vi "Log_File_Edits.vi"(0 "Job Directory":path=path "/G4_2_HD/Users/paulhayden/Documents/Projects/Hong Roughness/XW data/XW_Corr.tpt", 1 "File Editted?":bool, 2 "Channels to Edit":string[](array[string]), 3 "Data":string[][](array[string]), 4 "Results file name":path) -> ()   [LabVIEW 2011]
uses:
  Data_File_Type.ctl
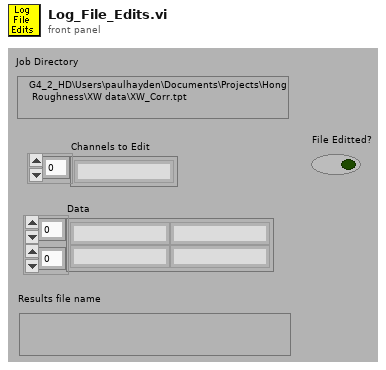
[diagram p1: front panel]
types:
  T1 = typedef "Data_File_Type.ctl" = enum16{"Read All File Types", "Results Files Only", "Raw Data Files Only", "Calibration Files Only", "Gas Desk Files Only", "Old Results Files Only", "Tabulated Data Files Only"}
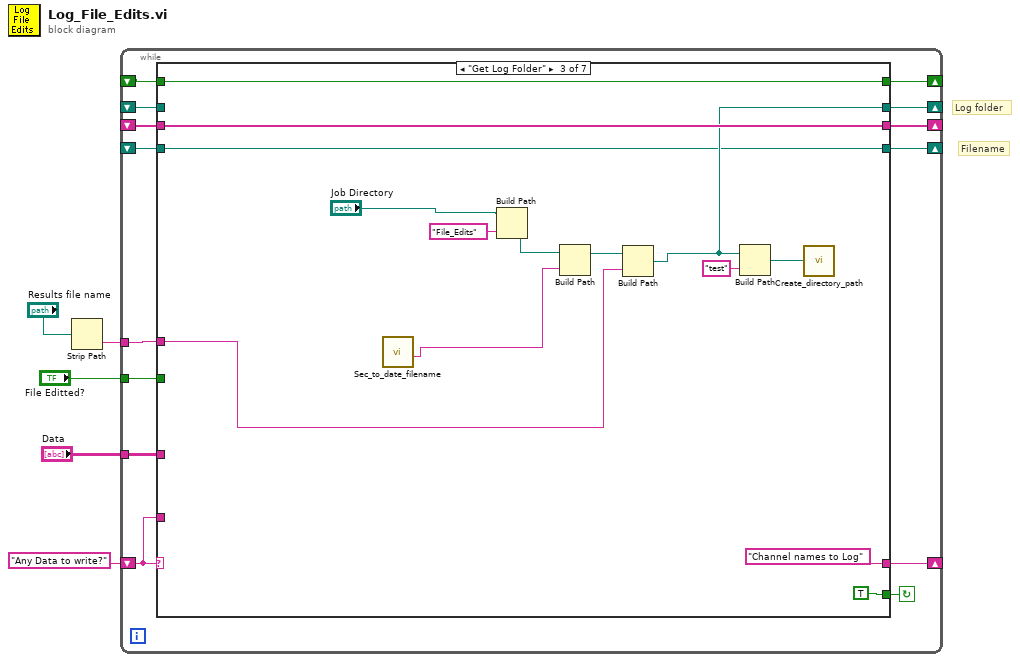
[diagram p0: block diagram]
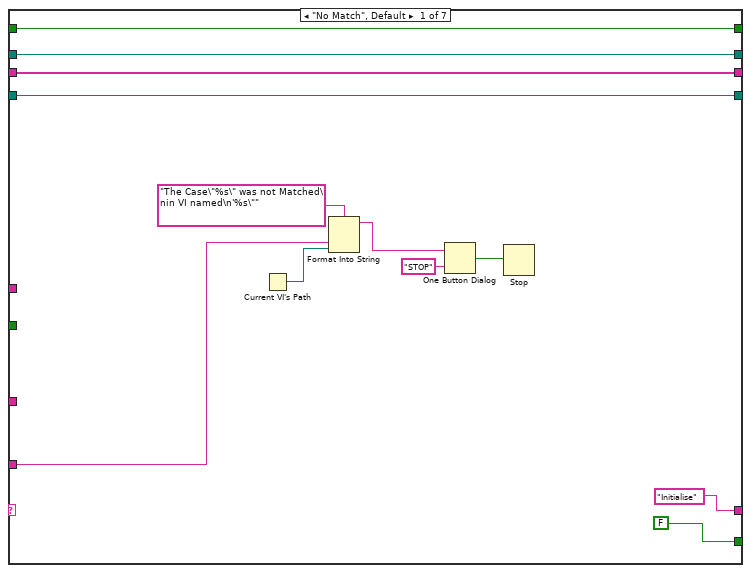
[diagram p2: hidden frame]
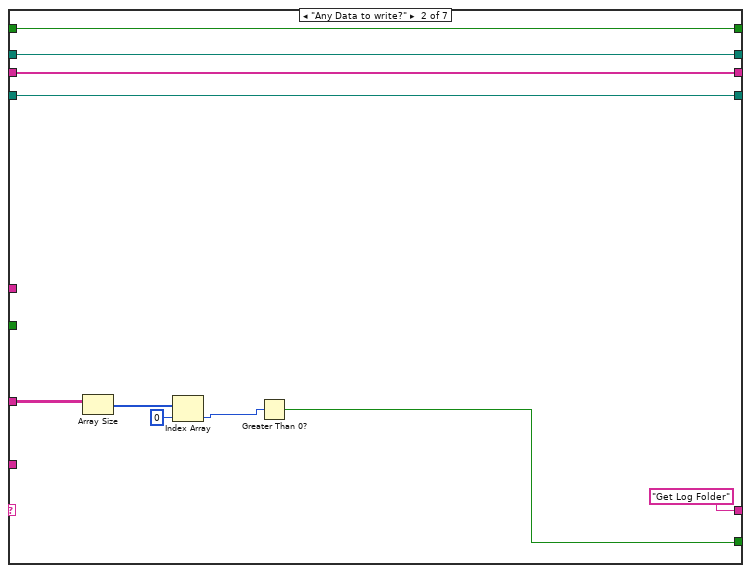
[diagram p3: hidden frame]
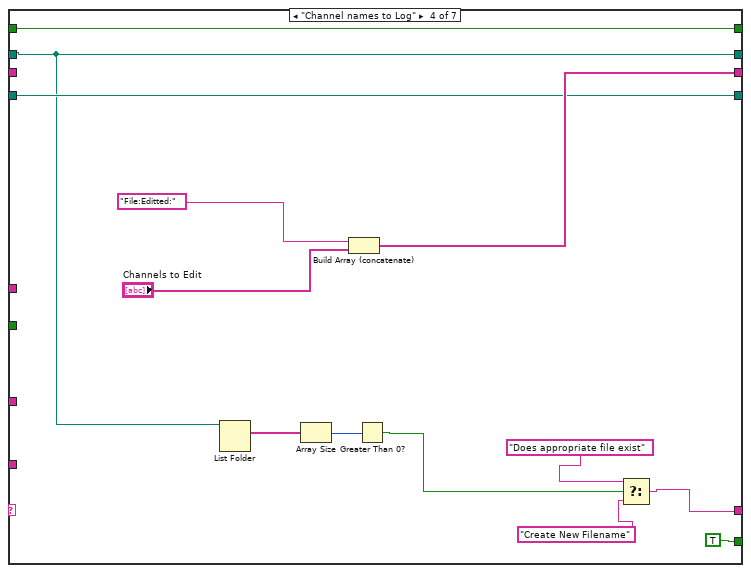
[diagram p4: hidden frame]
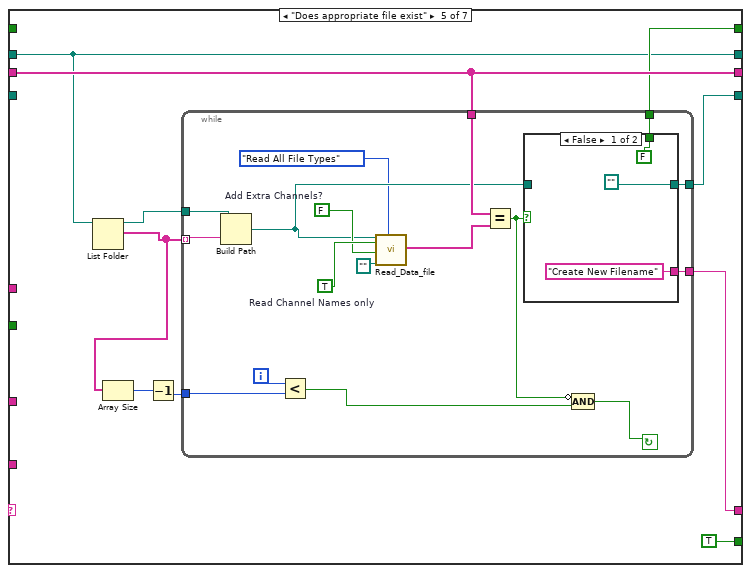
[diagram p5: hidden frame]
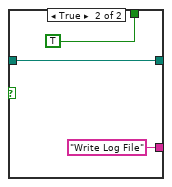
[diagram p6: hidden frame]
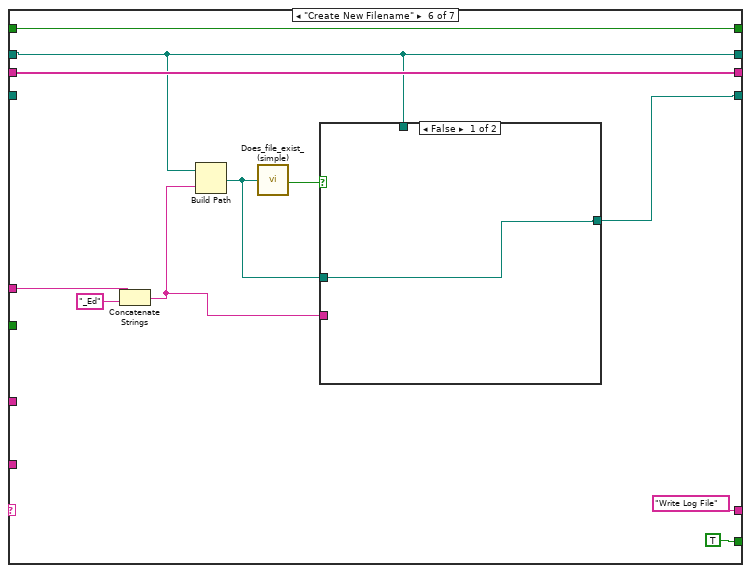
[diagram p7: hidden frame]
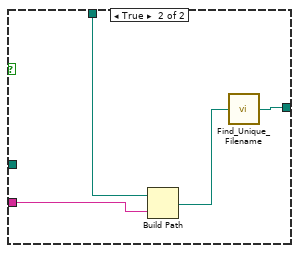
[diagram p8: hidden frame]
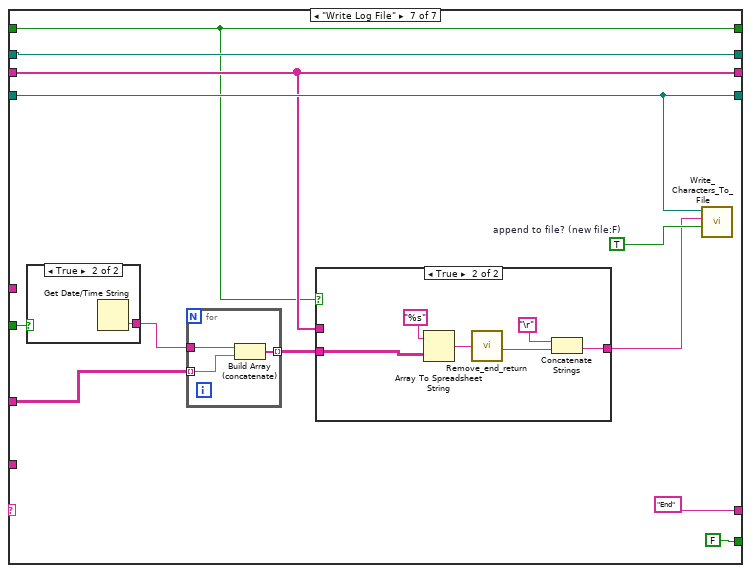
[diagram p9: hidden frame]
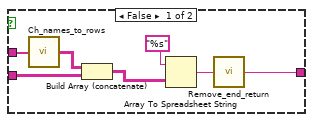
[diagram p10: hidden frame]
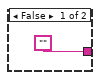
[diagram p11: hidden frame]
diagram:
  # "Filename"
  # "Log folder"
  n1 = Strip Path(path="Results file name") -> (name=w3:string)  [unwired: 1 out]
  n2 = while {
    shift-left: "Any Data to write?" -> [w17]
    shift-right: [w18] -> _
    shift-right: [w15] -> _
    shift-left: _ -> [w14]
    shift-right: [w16] -> _
    shift-left: _ -> [w13]
    tunnel: w3 -> [w12]
    shift-right: [w11] -> _
    shift-left: _ -> [w10]
    shift-right: [w9] -> _
    shift-left: _ -> [w8]
    tunnel: "File Editted?" -> [w7]
    tunnel: "Data" -> [w6]
    stop <- w19 continue-if-true
    n3 = case shown="\"Get Log Folder\"" w17 {
      tunnel: [FALSE w32 TRUE TRUE TRUE TRUE FALSE] -> w19
      tunnel: ["Initialise" "Get Log Folder" "Channel names to Log" w57 w71 "Write Log File" "End"] -> w18
      tunnel: w17 -> [w26 _ _ _ _ _ _]
      tunnel: w10 -> [w21 w38 w45 w65 _ _ w122]
      tunnel: [w22 w39 w51 w66 w76 w110 w121] -> w16
      tunnel: [w23 w40 w47 w62 w69 w104 w127] -> w15
      tunnel: w14 -> [w23 w40 _ w62 w69 w104 w127]
      tunnel: w13 -> [w22 w39 w51 _ w76 w110 w121]
      tunnel: w12 -> [_ _ w46 _ _ w103 _]
      tunnel: [w21 w38 w45 w65 w74 w108 w122] -> w11
      tunnel: [w20 w37 w44 w64 w70 w107 w119] -> w9
      tunnel: w8 -> [w20 w37 w44 w64 _ w107 w119]
      tunnel: w7 -> [_ _ _ _ _ _ w124]
      tunnel: w6 -> [_ w36 _ _ _ _ w118]
      frame "No Match", Default {
        n4 = Current VI's Path() -> (path=w25:path)
        n5 = Format Into String(format string="The Case\"%s\" was not Matched\nin VI named\n'%s\"" ("Format String"), w26, w25) -> (resulting string=w29:string)  [unwired: 2 in, 1 out]
        n6 = One Button Dialog(message=w29, button name ("OK")="STOP") -> (true=w27:bool)
        n7 = Stop(stop? (T)=w27) -> ()
      }
      frame "Any Data to write?" {
        n8 = Array Size(array=w36) -> (size(s)=w35:i32[])
        n9 = Index Array(array=w35, index=0) -> (element=w33:i32)
        n10 = Greater Than 0?(x=w33) -> (x > 0?=w32:bool)
      }
      frame "Get Log Folder" {
        n11 = call "Sec_to_date_filename.vi"() -> ("Day"=w42:string)  [unwired: 1 in, 3 out]
        n12 = Build Path(base path="Job Directory", name or relative path="File_Edits") -> (appended path=w49:path)
        n13 = Build Path(base path=w49, name or relative path=w42) -> (appended path=w48:path)
        n14 = Build Path(base path=w48, name or relative path=w46) -> (appended path=w47:path)
        n15 = Build Path(base path=w47, name or relative path="test") -> (appended path=w52:path)
        n16 = call "Create_directory_path.vi"("Path name"=w52) -> ()  [unwired: 1 in, 2 out]
      }
      frame "Channel names to Log" {
        n17 = List Folder(path=w62) -> (filenames=w61:string[])  [unwired: 1 in, 5 out]
        n18 = Array Size(array=w61) -> (size(s)=w60:i32)
        n19 = Build Array (concatenate)("File:Editted:", "Channels to Edit") -> (w66:string[])
        n20 = Greater Than 0?(x=w60) -> (x > 0?=w59:bool)
        n21 = Select(t="Does appropriate file exist", s=w59, f="Create New Filename") -> (s? t:f=w57:string)
      }
      frame "Does appropriate file exist" {
        n22 = List Folder(path=w69) -> (path out=w77:path, filenames=w75:string[])  [unwired: 1 in, 4 out]
        n23 = Array Size(array=w75) -> (size(s)=w73:i32)
        n24 = Decrement(x=w73) -> (x-1=w72:i32)
        n25 = while {
          tunnel: w75 -> [w94] mode=indexing
          tunnel: w77 -> [w95]
          tunnel: w76 -> [w89]
          tunnel: [w88] -> w74
          tunnel: w72 -> [w85]
          tunnel: [w81] -> w71
          tunnel: [w80] -> w70
          i -> [w86]
          stop <- w82 continue-if-true
          w92 = FALSE  # Add Extra Channels?
          w93 = TRUE  # Read Channel Names only
          n26 = Build Path(base path=w95, name or relative path=w94) -> (appended path=w87:path)
          n27 = Less?(x=w86, y=w85) -> (x < y?=w84:bool)
          n28 = call "Read_Data_file.vi"("Results file"=w87, "Read Channel Names only"=w93, "Add Extra Channels?"=w92, "Template File"=path "", "Desired File Types"=Data_File_Type."Read All File Types") -> ("Ch names Out"=w90:string[])  [unwired: 14 out]
          n29 = Equal?(x=w89, y=w90) -> (x = y?=w83:bool)
          n30 = case shown="False" w83 {
            tunnel: [path "" w101] -> w88
            tunnel: w87 -> [_ w101]
            tunnel: ["Create New Filename" "Write Log File"] -> w81
            tunnel: [FALSE TRUE] -> w80
            frame False {
            }
            frame True {
            }
          }
          n31 = Compound Arithmetic op=AND(invert w83, w84) -> (w82:bool)
        }
      }
      frame "Create New Filename" {
        n32 = Concatenate Strings(w103, "_Ed" ("string")) -> (w102:string)
        n33 = Build Path(base path=w104, name or relative path=w102) -> (appended path=w105:path)
        n34 = call "Does_file_exist_(simple).vi"("Pathname"=w105) -> ("exists?"=w106:bool)
        n35 = case shown="False" w106 {
          tunnel: [w113 w117] -> w108
          tunnel: w105 -> [w113 _]
          tunnel: w104 -> [_ w116]
          tunnel: w102 -> [_ w114]
          frame False {
          }
          frame True {
            n36 = Build Path(base path=w116, name or relative path=w114) -> (appended path=w115:path)
            n37 = call "Find_Unique_Filename.vi"("Path In"=w115) -> ("Unique Path Out"=w117:path)  [unwired: 1 in, 1 out]
          }
        }
      }
      frame "Write Log File" {
        w126 = TRUE  # append to file? (new file:F)
        n38 = case shown="True" w124 {
          tunnel: ["" w144] -> w125
          frame False {
          }
          frame True {
            n39 = Get Date/Time String() -> (time string=w144:string)  [unwired: 4 out]
          }
        }
        n40 = for {
          tunnel: w118 -> [w147] mode=indexing
          tunnel: w125 -> [w146]
          tunnel: [w145] -> w120 mode=indexing
          n41 = Build Array (concatenate)(w146, w147) -> (w145:string[])
        }
        n42 = case shown="True" w119 {
          tunnel: [w134 w138] -> w123
          tunnel: w121 -> [w132 _]
          tunnel: w120 -> [w131 w140]
          frame False {
            n43 = call "Ch_names_to_rows.vi"("Channel Names"=w132) -> ("3 Row names"=w133:string[][])
            n44 = Build Array (concatenate)(w133, w131) -> (w130:string[][])
            n45 = Array To Spreadsheet String(array=w130, 3:"%s" ("format string")) -> (spreadsheet string=w136:string)  [unwired: 1 out]
            n46 = call "Remove_end_return.vi"("Input string"=w136) -> ("Output string"=w134:string)
          }
          frame True {
            n47 = Array To Spreadsheet String(array=w140, 3:"%s" ("format string")) -> (spreadsheet string=w142:string)  [unwired: 1 out]
            n48 = call "Remove_end_return.vi"("Input string"=w142) -> ("Output string"=w139:string)
            n49 = Concatenate Strings("\r", w139) -> (w138:string)
          }
        }
        n50 = call "Write_Characters_To_File.vi"("file path (dialog if empty)"=w122, "character string"=w123, "append to file? (new file:F)"=w126) -> ()  [unwired: 2 in, 4 out]
      }
    }
  }
